vi "_Parse Detected Modulation.vi"(8 "error in (no error)":errorcluster, 10 "Input String":string, 11 "VISA resource name":refnum<visa-resource-name>) -> (0 "error out":errorcluster, 1 "Result":i32, 2 "Reliability":i32, 3 "VISA resource name out":refnum<visa-resource-name>)   [LabVIEW 2020, in "Rohde&Schwarz CMXP NR FR2 Measurement.lvlib"]
uses:
  <instrlib>/Rohde&Schwarz CMXP NR FR2 Measurement/Rohde&Schwarz CMXP NR FR2 Measurement.lvlib
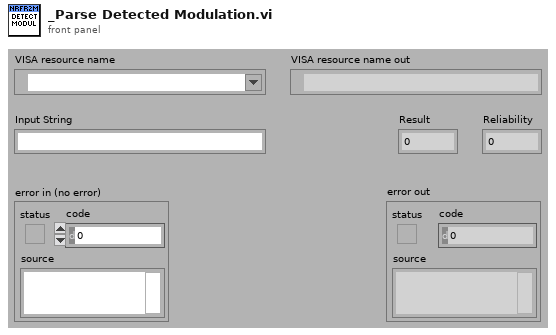
[diagram p1: front panel]
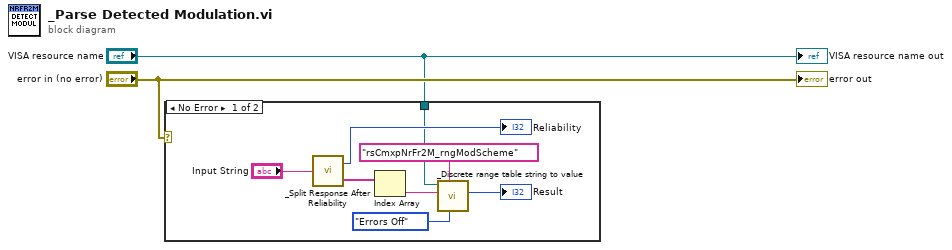
[diagram p0: block diagram]
diagram:
  n1 = case shown="No Error" "error in (no error)" {
    tunnel: "VISA resource name" -> [w3 _]
    frame No Error {
      n2 = call <instrlib>:"_Split Response After Reliability.vi"("Input String"="Input String") -> ("Response out"=w8:string[], "Reliability out"=→"Reliability":i32)
      n3 = Index Array(array=w8) -> (element=w7:string)  [unwired: 1 in]
      n4 = call <instrlib>:"_Discrete range table string to value.vi"("Error Mode (Warnings)"=enum16{"Errors Off", "Errors", "Warnings"}."Errors Off", "Discrete Range Table Identifier"="rsCmxpNrFr2M_rngModScheme", "String Value In"=w7, "VISA resource name"=w3) -> ("Enum Value"=→"Result":i32)  [unwired: 5 in, 2 out]
    }
    frame Error {
    }
  }
  "VISA resource name out" <- "VISA resource name"
  "error out" <- "error in (no error)"
